vi "Exchange ALR_ON_OFFs.vi"(8 "error in (no error)":errorcluster, 9 "modified (0)":u16, 10 "ALR_ON_OFF":T1, 11 "ALR_ON_OFF_DVR":refnum<data-value>) -> (0 "error out":errorcluster, 2 "ALR_ON_OFF out":T1, 3 "ALR_ON_OFF out":refnum<data-value>)   [LabVIEW 2019, in "Alarms.lvlib"]
uses:
  Alarms.lvlib
  Ctl/ALR_ON_OFF.ctl
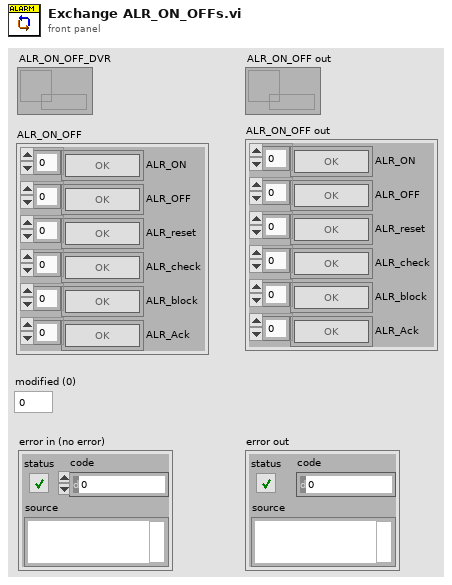
[diagram p1: front panel]
types:
  T1 = typedef "Alarms.lvlib/ALR_ON_OFF.ctl" = cluster{"ALR_ON":bool[], "ALR_OFF":bool[], "ALR_reset":bool[], "ALR_check":bool[], "ALR_block":bool[], "ALR_Ack":bool[]}
  T2 = cluster{"ALR_ON":bool[], "ALR_OFF":bool[], "ALR_reset":bool[], "ALR_check":bool[], "ALR_block":bool[], "ALR_Ack":bool[]}
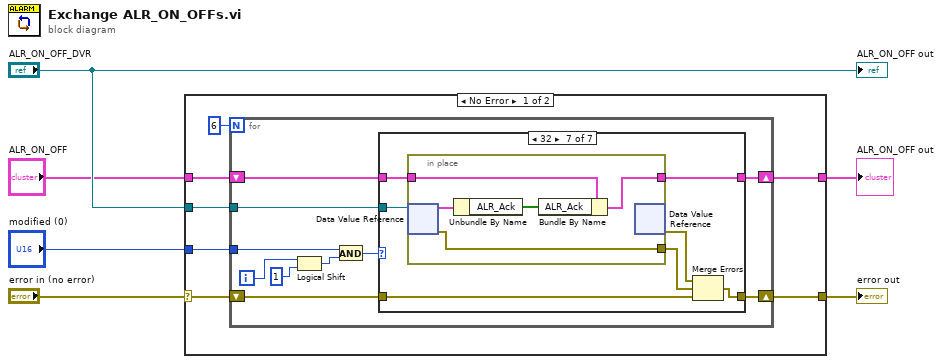
[diagram p0: block diagram]
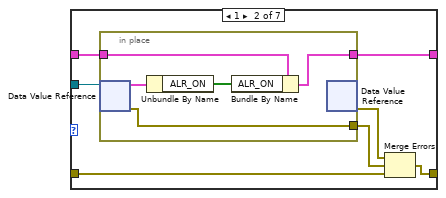
[diagram p3: hidden frame]
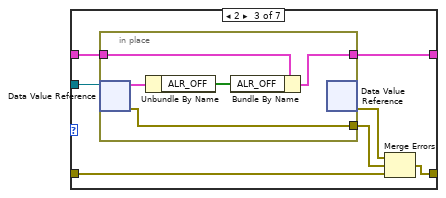
[diagram p4: hidden frame]
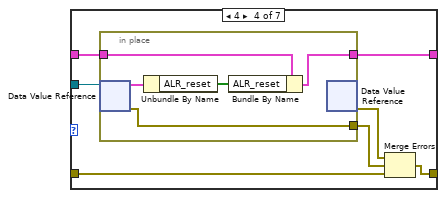
[diagram p5: hidden frame]
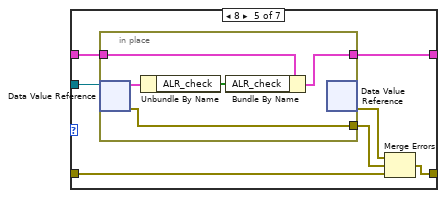
[diagram p6: hidden frame]
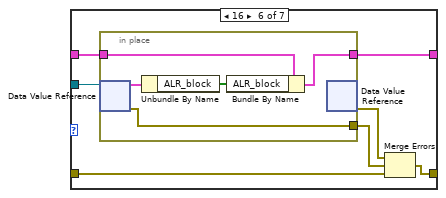
[diagram p7: hidden frame]
diagram:
  n1 = case shown="No Error" "error in (no error)" {
    selector: "error in (no error)" -> [w9 w99]
    tunnel: [w12 w99] -> w5
    tunnel: "ALR_ON_OFF_DVR" -> [w13 _]
    tunnel: "modified (0)" -> [w11 _]
    tunnel: "ALR_ON_OFF" -> [w10 w98]
    tunnel: [w8 w98] -> w1
    frame No Error {
      n2 = for {
        N: 6 -> [_]
        tunnel: w13 -> [w23]
        tunnel: w11 -> [w17]
        shift-right: [w15] -> w8
        shift-left: w10 -> [w19]
        shift-right: [w22] -> w12
        shift-left: w9 -> [w14]
        i -> [w21]
        n3 = Logical Shift(y=w21, x=u8 1 ("y")) -> (x << y=w16:u8)
        n4 = And(x=w17, y=w16) -> (x .and. y?=w20:u16)
        n5 = case shown="32" w20 {
          tunnel: w23 -> [_ w32 w44 w56 w68 w80 w92]
          tunnel: [w24 w29 w41 w53 w65 w77 w89] -> w22
          tunnel: w19 -> [w25 w28 w40 w52 w64 w76 w88]
          tunnel: [w25 w27 w39 w51 w63 w75 w87] -> w15
          tunnel: w14 -> [w24 w26 w38 w50 w62 w74 w86]
          frame 0, Default {
          }
          frame 1 {
            n6 = in-place {
              in-place-border: [w36] -> w30
              in-place-border: w28 -> [w35]
              in-place-border: [w34] -> w27
              n7 = in-place-dvr #1(w32) -> (w37:T2, w36:errorcluster)
              n8 = Unbundle By Name(w37) -> ("ALR_ON"=w33:bool[])
              n9 = Bundle By Name(cluster=w35, "ALR_ON"=w33) -> (w34:T1)
              n10 = in-place-dvr #1() -> (w31:errorcluster)  [unwired: 1 in, 1 out]
            }
            n11 = Merge Errors(w31, w30, w26) -> (w29:errorcluster)
          }
          frame 2 {
            n12 = in-place {
              in-place-border: [w48] -> w42
              in-place-border: w40 -> [w47]
              in-place-border: [w46] -> w39
              n13 = in-place-dvr #2(w44) -> (w49:T2, w48:errorcluster)
              n14 = Unbundle By Name(w49) -> ("ALR_OFF"=w45:bool[])
              n15 = Bundle By Name(cluster=w47, "ALR_OFF"=w45) -> (w46:T1)
              n16 = in-place-dvr #2() -> (w43:errorcluster)  [unwired: 1 in, 1 out]
            }
            n17 = Merge Errors(w43, w42, w38) -> (w41:errorcluster)
          }
          frame 4 {
            n18 = in-place {
              in-place-border: [w60] -> w54
              in-place-border: w52 -> [w59]
              in-place-border: [w58] -> w51
              n19 = in-place-dvr #3(w56) -> (w61:T2, w60:errorcluster)
              n20 = Unbundle By Name(w61) -> ("ALR_reset"=w57:bool[])
              n21 = Bundle By Name(cluster=w59, "ALR_reset"=w57) -> (w58:T1)
              n22 = in-place-dvr #3() -> (w55:errorcluster)  [unwired: 1 in, 1 out]
            }
            n23 = Merge Errors(w55, w54, w50) -> (w53:errorcluster)
          }
          frame 8 {
            n24 = in-place {
              in-place-border: [w72] -> w66
              in-place-border: w64 -> [w71]
              in-place-border: [w70] -> w63
              n25 = in-place-dvr #4(w68) -> (w73:T2, w72:errorcluster)
              n26 = Unbundle By Name(w73) -> ("ALR_check"=w69:bool[])
              n27 = Bundle By Name(cluster=w71, "ALR_check"=w69) -> (w70:T1)
              n28 = in-place-dvr #4() -> (w67:errorcluster)  [unwired: 1 in, 1 out]
            }
            n29 = Merge Errors(w67, w66, w62) -> (w65:errorcluster)
          }
          frame 16 {
            n30 = in-place {
              in-place-border: [w84] -> w78
              in-place-border: w76 -> [w83]
              in-place-border: [w82] -> w75
              n31 = in-place-dvr #5(w80) -> (w85:T2, w84:errorcluster)
              n32 = Unbundle By Name(w85) -> ("ALR_block"=w81:bool[])
              n33 = Bundle By Name(cluster=w83, "ALR_block"=w81) -> (w82:T1)
              n34 = in-place-dvr #5() -> (w79:errorcluster)  [unwired: 1 in, 1 out]
            }
            n35 = Merge Errors(w79, w78, w74) -> (w77:errorcluster)
          }
          frame 32 {
            n36 = in-place {
              in-place-border: [w96] -> w90
              in-place-border: w88 -> [w95]
              in-place-border: [w94] -> w87
              n37 = in-place-dvr #6(w92) -> (w97:T2, w96:errorcluster)
              n38 = Unbundle By Name(w97) -> ("ALR_Ack"=w93:bool[])
              n39 = Bundle By Name(cluster=w95, "ALR_Ack"=w93) -> (w94:T1)
              n40 = in-place-dvr #6() -> (w91:errorcluster)  [unwired: 1 in, 1 out]
            }
            n41 = Merge Errors(w91, w90, w86) -> (w89:errorcluster)
          }
        }
      }
    }
    frame Error {
    }
  }
  "error out" <- w5
  "ALR_ON_OFF out" <- w1
  "ALR_ON_OFF out" <- "ALR_ON_OFF_DVR"
